vi "Create Scheduler.vi"(8 "error in (no error)":errorcluster, 10 "Plugins":refnum<class "Plugin.lvclass">[](array[class]), 11 "Framework in":refnum<class "Framework.lvclass">) -> (0 "error out":errorcluster, 3 "Framework out":refnum<class "Framework.lvclass">)   [LabVIEW 2017, in "DSF Core.lvlib" / "Framework.lvclass"]
uses:
  Framework.lvclass
  Plugin/Plugin.lvclass
  Framework.lvclass/Framework.ctl
  Scheduler/Scheduler.lvclass
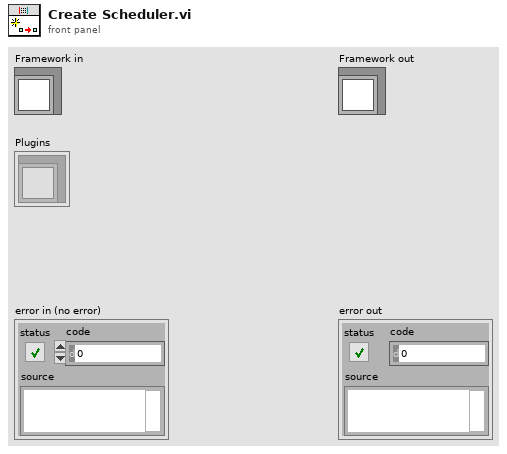
[diagram p1: front panel]
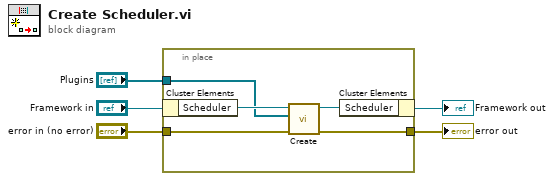
[diagram p0: block diagram]
diagram:
  n1 = in-place {
    in-place-border: "Plugins" -> [w8]
    in-place-border: "error in (no error)" -> [w6]
    in-place-border: [w7] -> w2
    n2 = in-place-cluster #1("Framework in") -> ("Scheduler"=w10:refnum<class "Scheduler.lvclass">)
    n3 = call "Create.vi"("error in (no error)"=w6, "Plugins"=w8, "Scheduler type"=w10) -> ("error out"=w7:errorcluster, "Scheduler"=w9:refnum<class "Scheduler.lvclass">)  [unwired: 7 in]
    n4 = in-place-cluster #1("Scheduler"=w9) -> (→"Framework out":refnum<class "Framework.lvclass">)
  }
  "error out" <- w2
